vi "一维布朗运动+改进？？统计直方图.vi"() -> ()   [LabVIEW 2017]
panel:
  out "移动次数":dbl
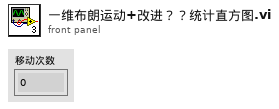
[diagram p1: front panel]
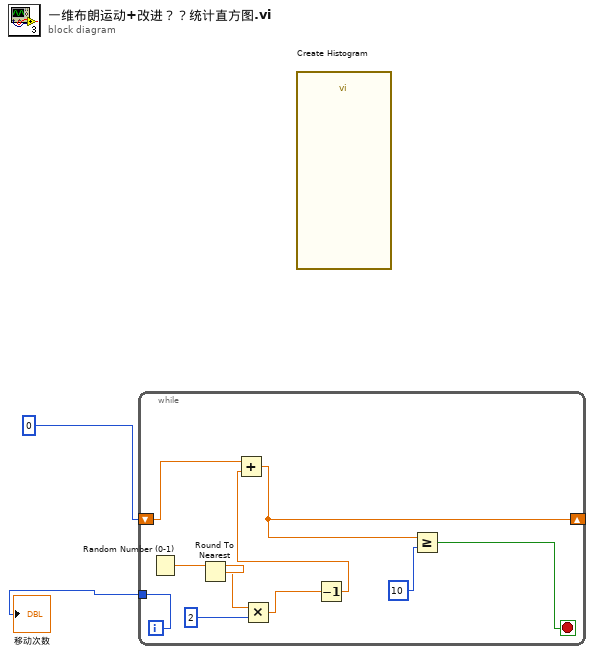
[diagram p0: block diagram]
diagram:
  n1 = while {
    shift-right: [w8] -> _
    shift-left: 0 -> [w10]
    tunnel: [w7] -> w1
    i -> [w7]
    stop <- w12 stop-if-true
    n2 = Random Number (0-1)() -> (number: 0 to 1=w6:dbl)
    n3 = Round To Nearest(number=w6) -> (nearest integer value=w4:dbl)
    n4 = Multiply(x=w4, y=2) -> (x*y=w3:dbl)
    n5 = Decrement(x=w3) -> (x-1=w11:dbl)
    n6 = Add(x=w10, y=w11) -> (x+y=w8:dbl)
    n7 = Greater Or Equal?(x=w8, y=10) -> (x >= y?=w12:bool)
  }
  "移动次数" <- w1
  n8 = call "Create Histogram"() -> ()  [unwired: 10 in, 2 out]
